vi "Queue.Reference.vi"(8 "error in (no error)":errorcluster, 11 "queueName":string) -> (0 "error out":errorcluster, 3 "refToQueue":refnum<queue>)   [LabVIEW 2019]
uses:
  QueueMessage.ctl
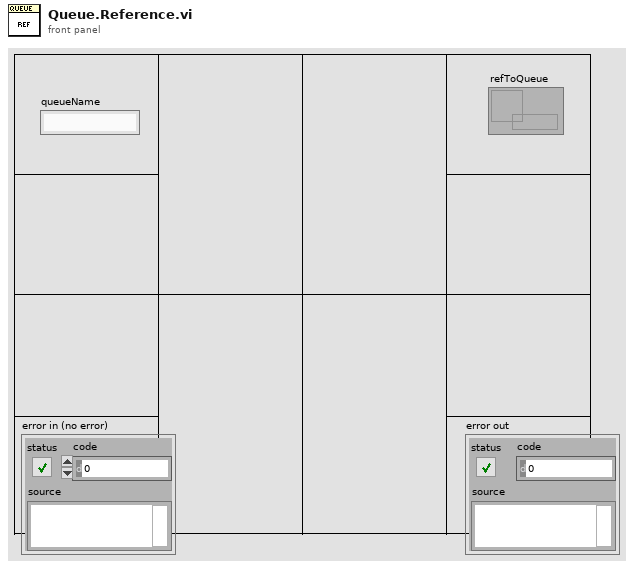
[diagram p1: front panel]
types:
  T1 = typedef "QueueMessage.ctl" = cluster{"message":string, "data":variant}
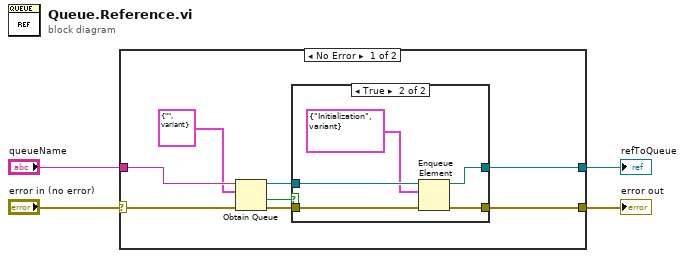
[diagram p0: block diagram]
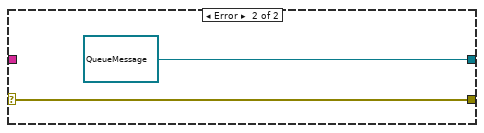
[diagram p3: hidden frame]
diagram:
  n1 = case shown="No Error" "error in (no error)" {
    selector: "error in (no error)" -> [w11 w21]
    tunnel: [w6 w21] -> w1
    tunnel: "queueName" -> [w12 _]
    tunnel: [w5 refnum<queue> refnum ("queue out")] -> w3
    frame No Error {
      n2 = Obtain Queue(name (unnamed)=w12, element data type=T1 {"message"="", "data"=variant} ("QueueMessage"), error in (no error)=w11) -> (queue out=w7:refnum<queue>, created new?=w9:bool, error out=w8:errorcluster)  [unwired: 2 in]
      n3 = case shown="True" w9 {
        tunnel: w8 -> [w14 w19]
        tunnel: w7 -> [w13 w18]
        tunnel: [w14 w17] -> w6
        tunnel: [w13 w16] -> w5
        frame False {
        }
        frame True {
          n4 = Enqueue Element(queue=w18, element=T1 {"message"="Initialization", "data"=variant} ("QueueMessage"), error in (no error)=w19) -> (queue out=w16:refnum<queue>, error out=w17:errorcluster)  [unwired: 1 in, 1 out]
        }
      }
    }
    frame Error {
    }
  }
  "refToQueue" <- w3
  "error out" <- w1
